vi "Write UI config file.vi"(8 "error in (no error)":errorcluster, 11 "?":T1={"Font"="Consolas", "Font Size"=0, "BG Color"=0, "Text Color"=0}) -> (0 "error out":errorcluster)   [LabVIEW 2023, in "VeriStand Console.lvlib"]
uses:
  VeriStand Console.lvlib
  TypeDefs/UI Settings.ctl
  <vilib>/Utility/config.llb/Write Key (String).vi
  <vilib>/Utility/config.llb/Write Key (U32).vi
  <vilib>/Utility/config.llb/NI_LVConfig.lvlib
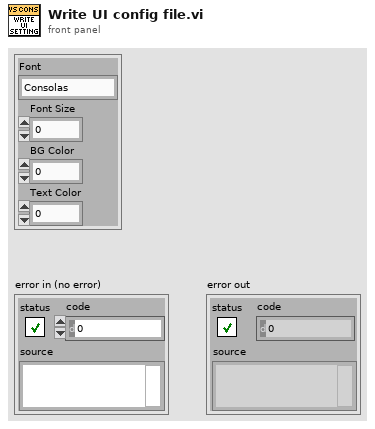
[diagram p1: front panel]
types:
  T1 = typedef "VeriStand Console.lvlib/UI Settings.ctl" = cluster{"Font":string, "Font Size":u32, "BG Color":u32, "Text Color":u32}
  T2 = typedef "NI_LVConfig.lvlib/Config Data RefNum.ctl" = refnum<k1>
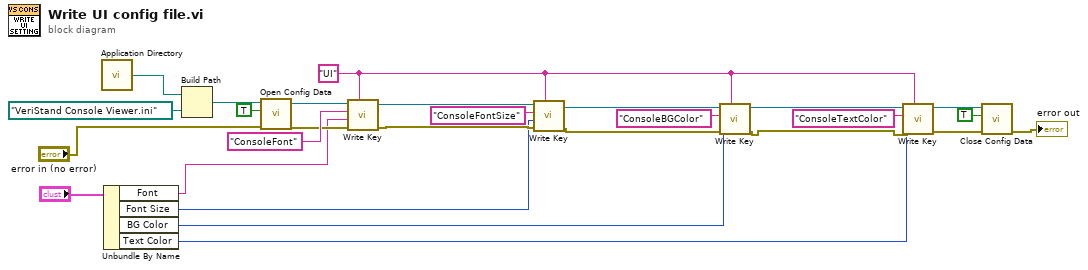
[diagram p0: block diagram]
diagram:
  w24 = "UI" ("section")
  n1 = call <vilib>:"Application Directory.vi"() -> ("Application Directory"=w11:path)
  n2 = Unbundle By Name("?") -> ("Font"=w9:string, "Font Size"=w8:u32, "BG Color"=w7:u32, "Text Color"=w6:u32)
  n3 = Build Path(base path=w11, name or relative path=path "VeriStand Console Viewer.ini") -> (appended path=w12:path)
  n4 = call <vilib>:"Open Config Data.vi"("error in (no error)"="error in (no error)", "create file if necessary (T)"=TRUE, "configuration file path"=w12) -> ("error out"=w16:errorcluster, "refnum"=w15:T2)  [unwired: 6 in, 1 out]
  n5 = call-poly <vilib>:"Write Key.vi"("section"=w24, "error in (no error)"=w16, "value"=w9, "key"="ConsoleFont", "refnum"=w15) -> ("error out"=w25:errorcluster, "refnum out"=w18:T2)  [unwired: 4 in, 1 out]
  n6 = call-poly <vilib>:"Write Key.vi"("section"=w24, "error in (no error)"=w25, "value"=w8, "key"="ConsoleFontSize", "refnum"=w18) -> ("error out"=w26:errorcluster, "refnum out"=w23:T2)  [unwired: 4 in, 1 out]
  n7 = call-poly <vilib>:"Write Key.vi"("section"=w24, "error in (no error)"=w26, "value"=w7, "key"="ConsoleBGColor", "refnum"=w23) -> ("error out"=w27:errorcluster, "refnum out"=w22:T2)  [unwired: 4 in, 1 out]
  n8 = call-poly <vilib>:"Write Key.vi"("section"=w24, "error in (no error)"=w27, "value"=w6, "key"="ConsoleTextColor", "refnum"=w22) -> ("error out"=w5:errorcluster, "refnum out"=w2:T2)  [unwired: 4 in, 1 out]
  n9 = call <vilib>:"Close Config Data.vi"("error in (no error)"=w5, "write file if changed (T)"=TRUE, "refnum"=w2) -> ("error out"=→"error out":errorcluster)  [unwired: 7 in, 1 out]
